vi "写入报告.vi"(6 "实测温度":dbl format="%#.3g", 8 "error in (no error)":errorcluster, 9 "目标温度":string, 10 "多通道温度值":dbl[](array[numeric]), 11 "report in":refnum<class "NI_report.lvclass">) -> (0 "error out":errorcluster)   [LabVIEW 2015]
uses:
  <vilib>/Utility/NIReport.llb/NI_report.lvclass
  <vilib>/Utility/NIReport.llb/Excel/NI_Excel.lvclass
  <vilib>/addons/_office/NI_ReportGenerationToolkit.lvlib
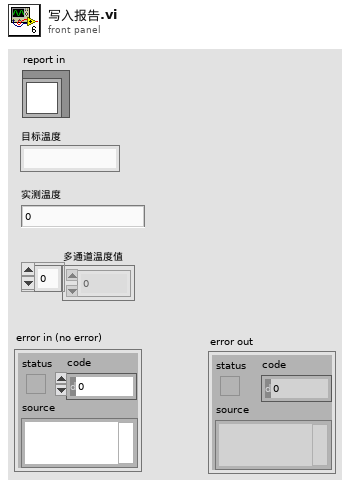
[diagram p1: front panel]
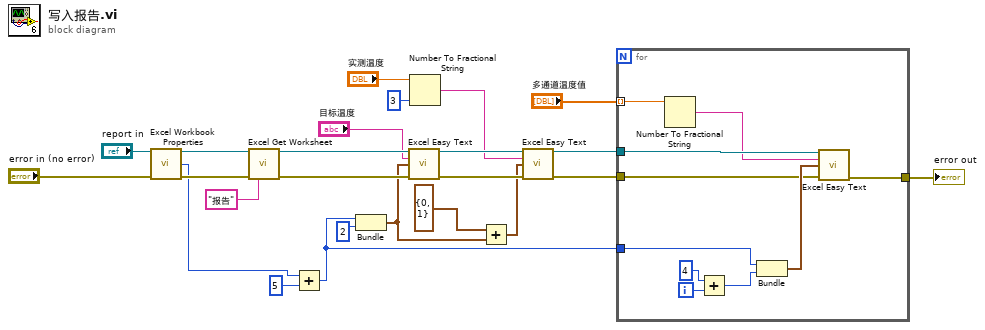
[diagram p0: block diagram]
diagram:
  n1 = call <vilib>:"Excel Workbook Properties.vi"("report in"="report in", "error in (no error)"="error in (no error)") -> ("report out"=w21:refnum<class "NI_report.lvclass">, "worksheets count"=w16:i32, "error out"=w20:errorcluster)  [unwired: 10 in, 1 out]
  n2 = call <vilib>:"Excel Get Worksheet.vi"("report in"=w21, "error in (no error)"=w20, "name (\"\")"="报告" ("name (\"\")")) -> ("report out"=w14:refnum<class "NI_report.lvclass">, "error out"=w15:errorcluster)  [unwired: 11 in]
  n3 = Add(x=w16, y=5) -> (x+y=w12:i32)
  n4 = Bundle(w12, "y"=2) -> (w3:cluster{i32, "y":i32})  [unwired: 1 in]
  n5 = call <vilib>:"Excel Easy Text.vi"("report in"=w14, "text"="目标温度", "start (-1, -1)"=w3, "error in (no error)"=w15) -> ("report out"=w9:refnum<class "NI_report.lvclass">, "error out"=w10:errorcluster)  [unwired: 7 in, 3 out]
  n6 = Number To Fractional String(number="实测温度", precision (6)=i16 3 ("精度(6)")) -> (F-format string=w4:string)  [unwired: 2 in]
  n7 = Add(x=cluster{"row":i32, "column":i32} {"row"=0, "column"=1} ("end (-1, -1)"), y=w3) -> (x+y=w1:cluster{i32, i32})
  n8 = call <vilib>:"Excel Easy Text.vi"("report in"=w9, "text"=w4, "start (-1, -1)"=w1, "error in (no error)"=w10) -> ("report out"=w7:refnum<class "NI_report.lvclass">, "error out"=w8:errorcluster)  [unwired: 7 in, 3 out]
  n9 = for {
    tunnel: w7 -> [w34]
    tunnel: "多通道温度值" -> [w33] mode=indexing
    tunnel: w8 -> [w27]
    tunnel: [w26] -> w18
    tunnel: w12 -> [w25]
    i -> [w31]
    n10 = Number To Fractional String(number=w33) -> (F-format string=w32:string)  [unwired: 3 in]
    n11 = Add(x=4 ("y"), y=w31) -> (x+y=w29:i32)
    n12 = Bundle(w25, w29) -> (w28:cluster{i32, i32})  [unwired: 1 in]
    n13 = call <vilib>:"Excel Easy Text.vi"("report in"=w34, "text"=w32, "start (-1, -1)"=w28, "error in (no error)"=w27) -> ("error out"=w26:errorcluster)  [unwired: 7 in, 4 out]
  }
  "error out" <- w18
